vi "Exists.vi"(8 "error in (no error)":errorcluster, 11 "Pointer Base in":refnum<class "Pointer Base.lvclass">) -> (0 "error out":errorcluster, 2 "exists?":bool, 3 "Pointer Base out":refnum<class "Pointer Base.lvclass">)   [LabVIEW 2020, in "PV Access.lvlib" / "Pointer Base.lvclass"]
uses:
  Pointer Base.lvclass
  Pointer Base.lvclass/Pointer Base.ctl
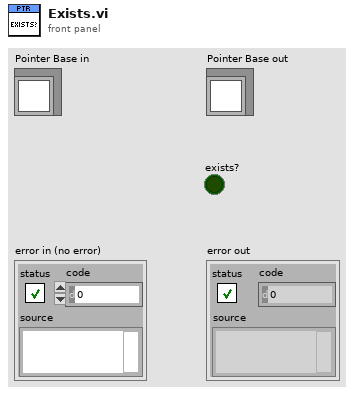
[diagram p1: front panel]
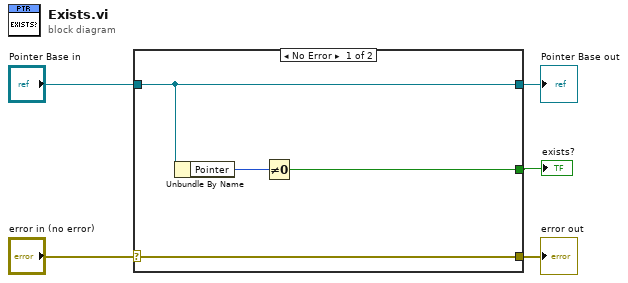
[diagram p0: block diagram]
diagram:
  n1 = case shown="No Error" "error in (no error)" {
    selector: "error in (no error)" -> [w9 w10]
    tunnel: [w9 w10] -> w4
    tunnel: [w8 w11] -> w2
    tunnel: "Pointer Base in" -> [w8 w11]
    tunnel: [w6 _] -> w1
    frame No Error {
      n2 = Unbundle By Name(w8) -> ("Pointer"=w7:i64)
      n3 = Not Equal To 0?(x=w7) -> (x != 0?=w6:bool)
    }
    frame Error {
    }
  }
  "error out" <- w4
  "Pointer Base out" <- w2
  "exists?" <- w1
